vi "boolean array to int array.vi"(11 "Array 3":bool[](array[boolean])) -> (2 "Array":bool[](array[boolean]), 3 "Array 2":u8[](array[numeric]))   [LabVIEW 2021]
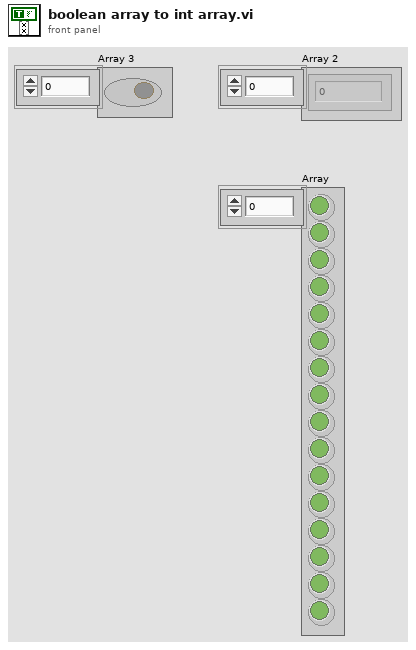
[diagram p1: front panel]
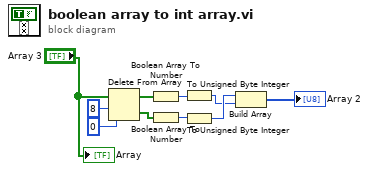
[diagram p0: block diagram]
diagram:
  n1 = Delete From Array(array="Array 3", length=8, index=0) -> (deleted portion=w5:bool[], array with subset deleted=w6:bool[])
  n2 = Boolean Array To Number(Boolean array=w6) -> (number=w4:u32)
  n3 = Boolean Array To Number(Boolean array=w5) -> (number=w3:u32)
  n4 = To Unsigned Byte Integer(number=w4) -> (unsigned 8bit integer=w1:u8)
  n5 = To Unsigned Byte Integer(number=w3) -> (unsigned 8bit integer=w2:u8)
  n6 = Build Array(w2, w1) -> (→"Array 2":u8[])
  "Array" <- "Array 3"
